vi "tuxing.vi"(0 "bean_x":dbl[](array[numeric]), 1 "xnew":dbl, 2 "ynew":dbl, 5 "bean_y":dbl[](array[numeric]), 9 "xy_in":cluster{"xi":dbl[], "yi":dbl[]}, 11 "map_in":cluster{"xi":dbl[], "yi":dbl[]}, 12 "n1":i32, 13 "n2":i32) -> (3 "XY Graph":cluster{"xi":dbl[], "yi":dbl[]}[](graph), 4 "a":dbl[](array[numeric]), 6 "b":dbl[](array[numeric]), 8 "pos_o":cluster{"xo":dbl[], "yo":dbl[]}, 10 "n1 2":i32, 15 "n2 2":i32)   [LabVIEW 2015]
uses:
  <vilib>/imath/engines/lvmath2/RunTimeEngine/Managers/WorkSpace/UID Generator.vi
  <vilib>/imath/engines/lvmath2/RunTimeEngine/IndexRead/NIMS V(S).vi
  <instcachedir>/0/NIMS V(S)_0488751826AF41519A22953C041130DC.lvgen/NIMS V(S)_0488751826AF41519A22953C041130DC_000.vi
  <vilib>/imath/engines/lvmath2/RunTimeEngine/RunTimeType/NIMS_RunTimeType_From StrictType (excl LVString).vi
  <instcachedir>/0/NIMS_RunTimeType_From StrictType (excl LVString)_EB1C38A9BC5048DA9ABDA8F781E54D21.lvgen/NIMS_RunTimeType_From StrictType (excl LVString)_EB1C38A9BC5048DA9ABDA8F781E54D21_000.vi
  <vilib>/imathl/engines/lvmath/Functions/Error Handling/Create Error.vi
  <vilib>/imath/engines/lvmath2/RunTimeEngine/LocalVariableDefStatement/MC_LocalVariableDefStatement_Display.vi
  <vilib>/imath/engines/lvmath2/RunTimeEngine/RangeToken/NIMS_Range_R2 - Integer.vi
  <instcachedir>/0/NIMS_Range_R2 - Integer_396D5D4FB869421F9245109A0975AD54.lvgen/NIMS_Range_R2 - Integer_396D5D4FB869421F9245109A0975AD54_000.vi
  <vilib>/imath/engines/lvmath2/RunTimeEngine/CommandStatement/MC_CommandStatement_break.vi
  <vilib>/imath/engines/lvmath2/RunTimeEngine/IndexReplace/NIMS V(S)=S.vi
  <instcachedir>/0/NIMS V(S)=S_9916D32195284AEB9D40BA9A64F3B0C5.lvgen/NIMS V(S)=S_9916D32195284AEB9D40BA9A64F3B0C5_000.vi
  <vilib>/imath/engines/lvmath2/RunTimeEngine/ErrorHandling/NIMS_Create Error From Enums.vi
  <vilib>/imath/engines/lvmath2/RunTimeEngine/Managers/SymbolTable/Clear UID.vi
  <vilib>/imath/engines/lvmath2/RunTimeEngine/NodeEndStatement/NIMS_NodeEndStatement_Output.vi
  <instcachedir>/0/NIMS_NodeEndStatement_Output_53EC0D466D134D7ABD903AC30B43404B.lvgen/NIMS_NodeEndStatement_Output_53EC0D466D134D7ABD903AC30B43404B_005.vi
  <vilib>/imath/engines/lvmath2/RunTimeEngine/ErrorHandling/NIMS_Finalize Error.vi
  <vilib>/imath/engines/lvmath2/RunTimeEngine/Managers/SymbolTable/NIMS_WorkSpace.lvlib
panel:
  out "b 3":dbl[](array[numeric])
  out "a 3":dbl[](array[numeric])
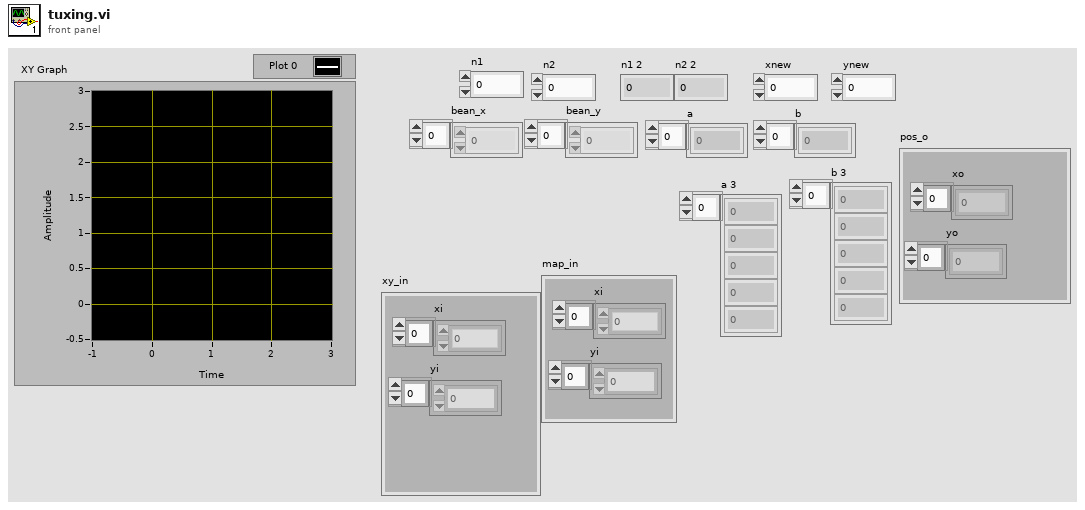
[diagram p1: front panel]
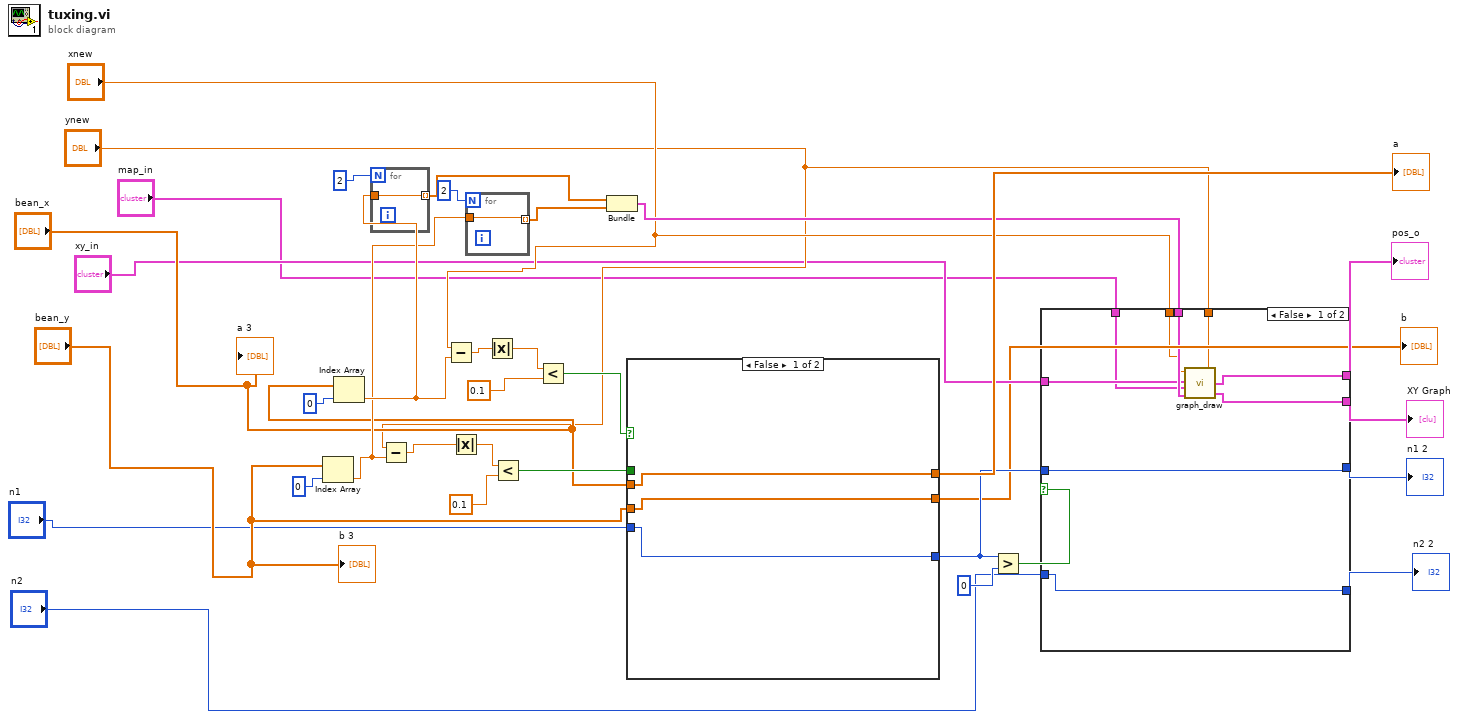
[diagram p0: block diagram]
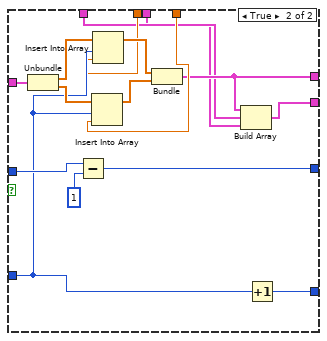
[diagram p2: hidden frame]
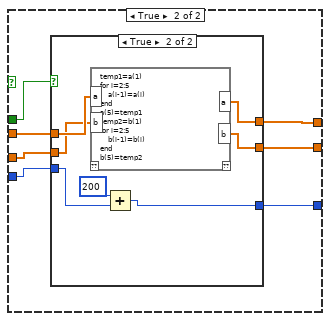
[diagram p3: hidden frame]
diagram:
  n1 = Index Array(array="bean_y", index=0) -> (element=w21:dbl)
  n2 = Index Array(array="bean_x", index=0) -> (element=w22:dbl)
  n3 = for {
    N: 2 -> [_]
    tunnel: w22 -> [w35]
    tunnel: [w35] -> w20 mode=indexing
  }
  n4 = Subtract(x="ynew", y=w21) -> (x-y=w31:dbl)
  n5 = Subtract(x="xnew", y=w22) -> (x-y=w32:dbl)
  n6 = Absolute Value(x=w31) -> (abs(x)=w30:dbl)
  n7 = for {
    N: 2 -> [_]
    tunnel: w21 -> [w36]
    tunnel: [w36] -> w19 mode=indexing
  }
  n8 = Absolute Value(x=w32) -> (abs(x)=w28:dbl)
  n9 = Less?(x=w30, y=0.1) -> (x < y?=w25:bool)
  n10 = Less?(x=w28, y=0.1) -> (x < y?=w26:bool)
  n11 = Bundle(w20, w19) -> (w12:cluster{dbl[], dbl[]})  [unwired: 1 in]
  n12 = case shown="False" w26 {
    tunnel: w25 -> [_ w46]
    tunnel: "bean_x" -> [w39 w45]
    tunnel: "bean_y" -> [w38 w44]
    tunnel: [w39 w43] -> w18
    tunnel: [w38 w42] -> w1
    tunnel: "n1" -> [w37 w41]
    tunnel: [w37 w40] -> w15
    frame False {
    }
    frame True {
      n13 = case shown="True" w46 {
        tunnel: w45 -> [w49 w56]
        tunnel: w44 -> [w48 w55]
        tunnel: [w49 w54] -> w43
        tunnel: [w48 w53] -> w42
        tunnel: w41 -> [w47 w52]
        tunnel: [w47 w50] -> w40
        frame False {
        }
        frame True {
          n14 = mathscript code="temp1=a(1)\nfor i=2:5\n    a(i-1)=a(i)\nend\na(5)=temp1\ntemp2=b(1)\nfor i=2:5\n    b(i-1)=b(i)\nend\nb(5)=temp2"("a"=w56, "b"=w55) -> ("a"=w54:dbl[], "b"=w53:dbl[])  [unwired: 1 in, 1 out]
          n15 = Add(x=200, y=w52) -> (x+y=w50:i32)
        }
      }
    }
  }
  "a" <- w18
  "b" <- w1
  n16 = Greater?(x=w15, y=0) -> (0:w16:bool)
  n17 = case shown="False" w16 {
    tunnel: w15 -> [w340 w356]
    tunnel: [w340 w354] -> w14
    tunnel: "n2" -> [w332 w347]
    tunnel: [w332 w353] -> w13
    tunnel: "xy_in" -> [w338 w352]
    tunnel: [w334 w344] -> w5
    tunnel: w12 -> [w339 w342]
    tunnel: "map_in" -> [w337 w343]
    tunnel: "xnew" -> [w336 w346]
    tunnel: "ynew" -> [w335 w345]
    tunnel: [w333 w341] -> w11
    frame False {
      n18 = call "graph_draw.vi"("yi"=w335, "element"=w339, "map_in"=w337, "xy_in"=w338, "xi"=w336) -> ("XY Graph"=w333:cluster{"xi":dbl[], "yi":dbl[]}[], "pos_o"=w334:cluster{"xo":dbl[], "yo":dbl[]})
    }
    frame True {
      n19 = Unbundle(w352) -> ("xi"=w351:dbl[], "yi"=w350:dbl[])
      n20 = Subtract(x=w356, y=1) -> (x-y=w354:i32)
      n21 = Insert Into Array(array=w350, index=w347, new element=w345) -> (w348:dbl[])
      n22 = Insert Into Array(array=w351, index=w347, new element=w346) -> (w349:dbl[])
      n23 = Bundle("xi"=w349, "yi"=w348) -> (w344:cluster{"xi":dbl[], "yi":dbl[]})  [unwired: 1 in]
      n24 = Build Array(w344, w343, w342) -> (w341:cluster{"xi":dbl[], "yi":dbl[]}[])
      n25 = Increment(x=w347) -> (x+1=w353:i32)
    }
  }
  "XY Graph" <- w11
  "n1 2" <- w14
  "n2 2" <- w13
  "pos_o" <- w5
  "a 3" <- "bean_x"
  "b 3" <- "bean_y"
